vi "2-6比较函数库与控件修饰.vi"() -> ()   [LabVIEW 2018]
panel:
  out "十六进制？":bool
  in  "字符":string
  out "x >= y?":bool
  in  "x":dbl
  in  "y":dbl
  out "s? t:f":dbl
  in  "选项卡控件":enum32{"选项卡 1", "选项卡 2", "选项卡 3"}(tab)
  in  "f":dbl
  in  "s":bool
  in  "t":dbl
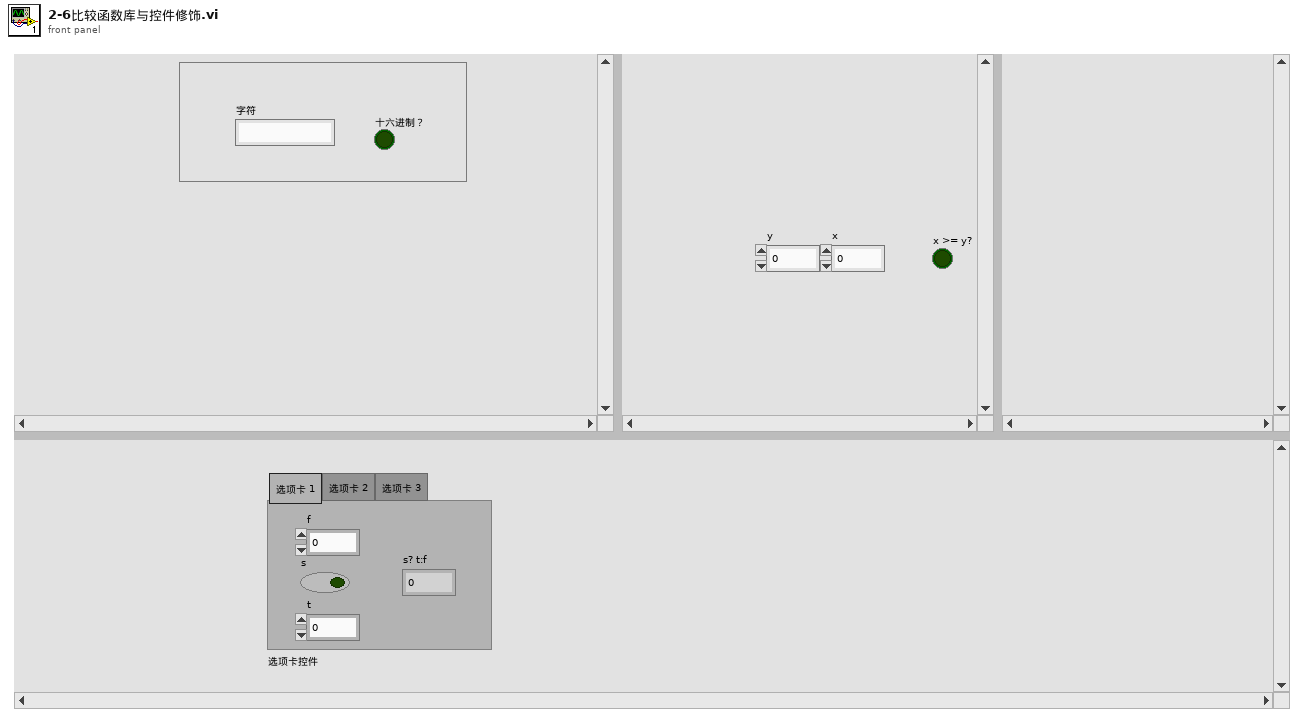
[diagram p1: front panel]
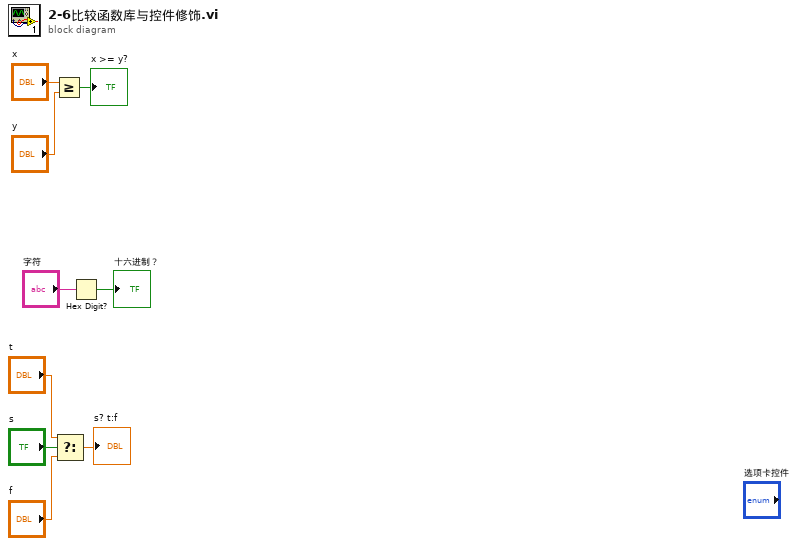
[diagram p0: block diagram]
diagram:
  n1 = Greater Or Equal?(x="x", y="y") -> (x >= y?=→"x >= y?":bool)
  n2 = Select(t="t", s="s", f="f") -> (s? t:f=→"s? t:f":dbl)
  n3 = Hex Digit?(1:"字符") -> (0:→"十六进制？":bool)
